vi "AT_Sequence_Select.vi"(9 "Array_Test":T1 {"Time to Wait (ms)" min=100; "ERD Number" format="%.0x"}, 10 "Sequence Select":T2) -> (2 "Array_Test_Out":T1 {"Time to Wait (ms)" min=100; "ERD Number" format="%.0x"})   [LabVIEW 2021]
uses:
  AT_Sequennce_Select.ctl
  AT_Erd_Sequence.ctl
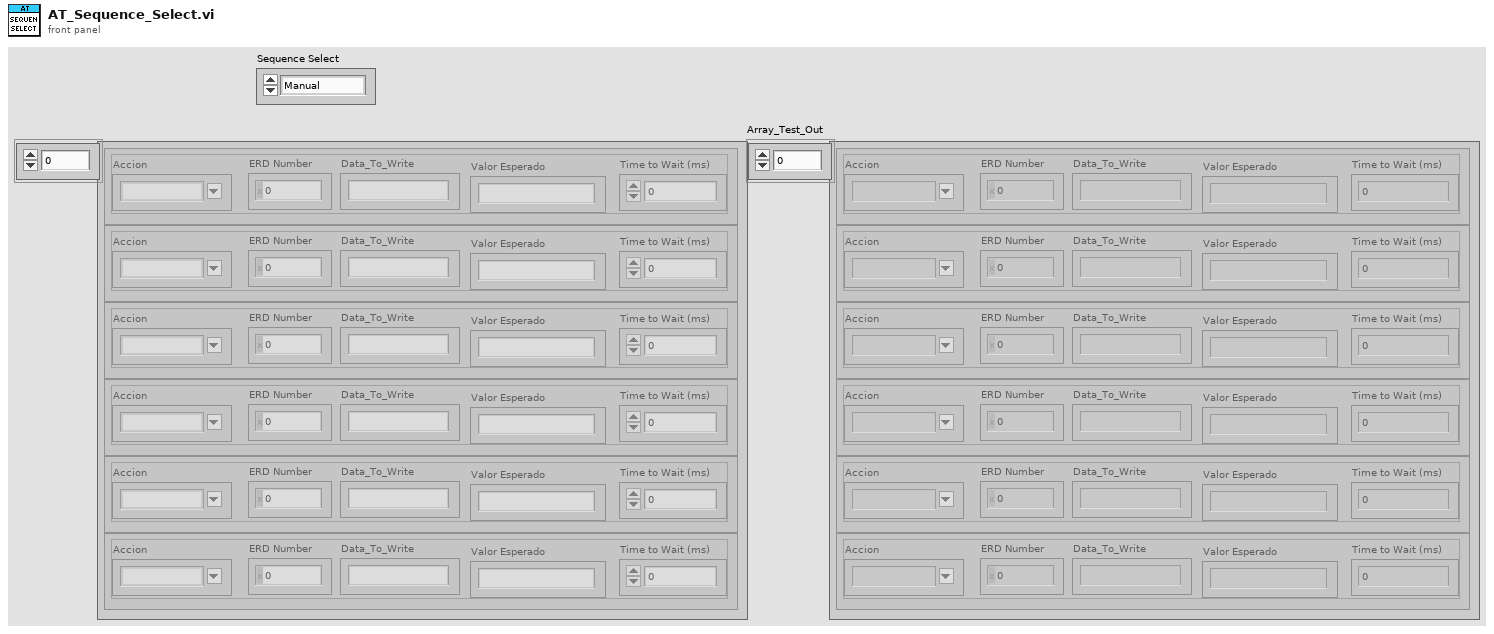
[diagram p1: front panel]
types:
  T1 = typedef "AT_Erd_Sequence.ctl" = cluster{"Accion":string, "Valor Esperado":string, "ERD Number":u16, "Data_To_Write":string, "Time to Wait (ms)":u32}[]
  T2 = typedef "AT_Sequennce_Select.ctl" = enum16{"Manual", "T346"}
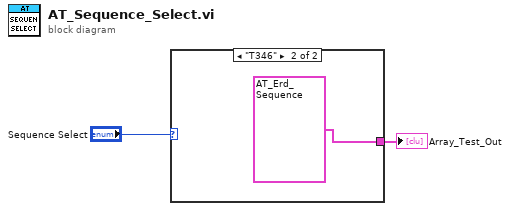
[diagram p0: block diagram]
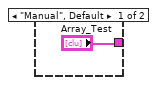
[diagram p2: hidden frame]
diagram:
  n1 = case shown="\"T346\"" "Sequence Select" {
    tunnel: ["Array_Test" T1 [{"Accion"="Leer", "Valor Esperado"="00", "ERD Number"=61548, "Data_To_Write"="", "Time to Wait (ms)"=0}, {"Accion"="Leer", "Valor Esperado"="00", "ERD Number"=61553, "Data_To_Write"="", "Time to Wait (ms)"=0}, {"Accion"="Leer", "Valor Esperado"="00", "ERD Number"=61546, "Data_To_Write"="", "Time to Wait (ms)"=1000}, {"Accion"="Leer", "Valor Esperado"="00", "ERD Number"=61547, "Data_To_Write"="", "Time to Wait (ms)"=0}, {"Accion"="Escribir", "Valor Esperado"="", "ERD Number"=61548, "Data_To_Write"="01", "Time to Wait (ms)"=0}, {"Accion"="Leer", "Valor Esperado"="00", "ERD Number"=61553, "Data_To_Write"="", "Time to Wait (ms)"=0}, {"Accion"="Escribir", "Valor Esperado"="", "ERD Number"=61546, "Data_To_Write"="04", "Time to Wait (ms)"=0}, {"Accion"="Leer", "Valor Esperado"="01", "ERD Number"=61548, "Data_To_Write"="", "Time to Wait (ms)"=0}, {"Accion"="Leer", "Valor Esperado"="01", "ERD Number"=61553, "Data_To_Write"="", "Time to Wait (ms)"=0}] ("T361")] -> w1
    frame "Manual", Default {
    }
    frame "T346" {
    }
  }
  "Array_Test_Out" <- w1
